vi "CloseOnDSClosed.vi"() -> (0 "Close?":bool)   [LabVIEW 2014]
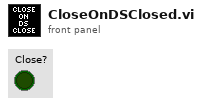
[diagram p1: front panel]
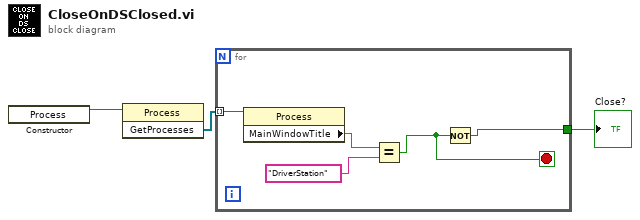
[diagram p0: block diagram]
diagram:
  n1 = constructor class="Process"() -> (reference out=w3:refnum<k24>)  [unwired: 3 in, 2 out]
  n2 = invoke class="Process" method="GetProcesses"(reference=w3) -> ("GetProcesses"=w1:refnum<k24>[])  [unwired: 2 in, 2 out]
  n3 = for {
    tunnel: w1 -> [w8] mode=indexing
    tunnel: [w5] -> w2
    stop <- w4 stop-if-true
    n4 = property class="Process"(reference=w8) -> ("MainWindowTitle"=w7:string)  [unwired: 1 in, 2 out]
    n5 = Equal?(x=w7, y="DriverStation") -> (x = y?=w4:bool)
    n6 = Not(x=w4) -> (.not. x?=w5:bool)
  }
  "Close?" <- w2
